vi "Initialize.vi"(8 "error in (no error)":errorcluster, 10 "Angle-Value Pairs":T1[](array[typedef]), 11 "LinearInterpolation in":refnum<class "LinearInterpolation.lvclass">) -> (0 "error out":errorcluster, 3 "LinearInterpolation out":refnum<class "LinearInterpolation.lvclass">)   [LabVIEW 2011, in "LinearInterpolation.lvclass"]
uses:
  LinearInterpolation.lvclass
  AngleValuePair.ctl
  LinearInterpolation.lvclass/LinearInterpolation.ctl
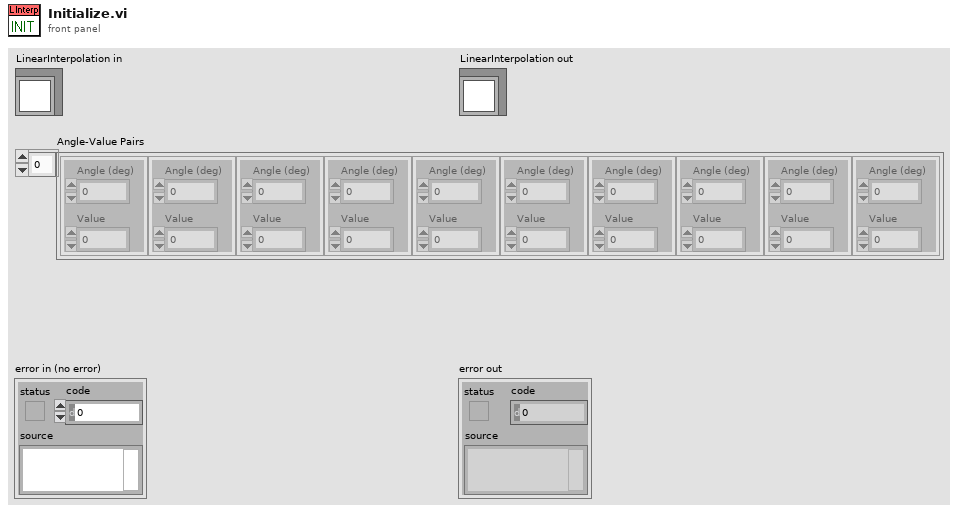
[diagram p1: front panel]
types:
  T1 = typedef "AngleValuePair.ctl" = cluster{"Angle (deg)":dbl, "Value":dbl}
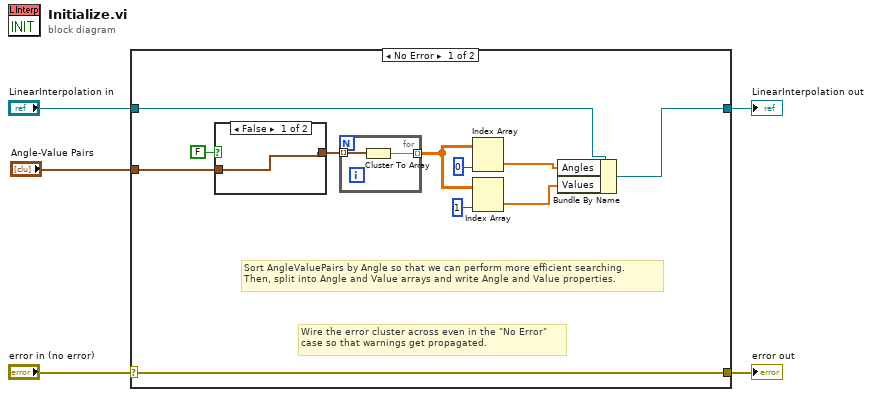
[diagram p0: block diagram]
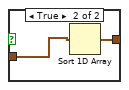
[diagram p2: hidden frame]
diagram:
  n1 = case shown="No Error" "error in (no error)" {
    selector: "error in (no error)" -> [w16 w23]
    tunnel: [w16 w23] -> w4
    tunnel: [w10 w22] -> w2
    tunnel: "LinearInterpolation in" -> [w11 w22]
    tunnel: "Angle-Value Pairs" -> [w9 _]
    frame No Error {
      # "Sort AngleValuePairs by Angle so that we can perform more efficient searching.\nThen, split into Angle and Value arrays and write Angle and Value properties."
      # "Wire the error cluster across even in the \"No Error\"\ncase so that warnings get propagated."
      n2 = case shown="False" FALSE {
        tunnel: [w17 w19] -> w15
        tunnel: w9 -> [w17 w18]
        frame False {
        }
        frame True {
          n3 = Sort 1D Array(array=w18) -> (sorted array=w19:T1[])
        }
      }
      n4 = for {
        tunnel: w15 -> [w20] mode=indexing
        tunnel: [w21] -> w12 mode=indexing
        n5 = Cluster To Array(cluster=w20) -> (array=w21:dbl[])
      }
      n6 = Index Array(array=w12, index (col)=0) -> (element=w8:dbl[])  [unwired: 1 in]
      n7 = Index Array(array=w12, index (col)=1) -> (element=w7:dbl[])  [unwired: 1 in]
      n8 = Bundle By Name(cluster=w11, "Angles"=w8, "Values"=w7) -> (w10:refnum<class "LinearInterpolation.lvclass">)
    }
    frame Error {
    }
  }
  "error out" <- w4
  "LinearInterpolation out" <- w2
